vi "TestLidar.vi"() -> ()   [LabVIEW 2018]
uses:
  <vilib>/robotics/Navigation/shared/MapNode/OccupancyGridNode/NI_Robotics_OccupancyGridMapNode.lvclass
  C:/Program Files (x86)/National Instruments/LabVIEW 2018/vi.lib/robotics/Navigation/shared/MapNode/AbstractAstarNode/NI_Robotics_AbstractAstarNode.lvclass
  <vilib>/robotics/Navigation/shared/WorldMap/OccupancyGridWorldMap/NI_Robotics_OccupancyGridWorldMap.lvclass
  C:/Program Files (x86)/National Instruments/LabVIEW 2018/vi.lib/robotics/Navigation/shared/WorldMap/AbstractWorldMap/NI_Robotics_AbstractWorldMap.lvclass
  <vilib>/robotics/Navigation/NI_Robotics_Navigation .lvlib
panel:
  out "Position (mm)":cluster{"X":dbl, "Y":dbl, "Theta":dbl}
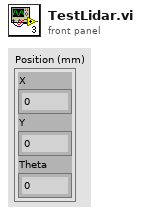
[diagram p1: front panel]
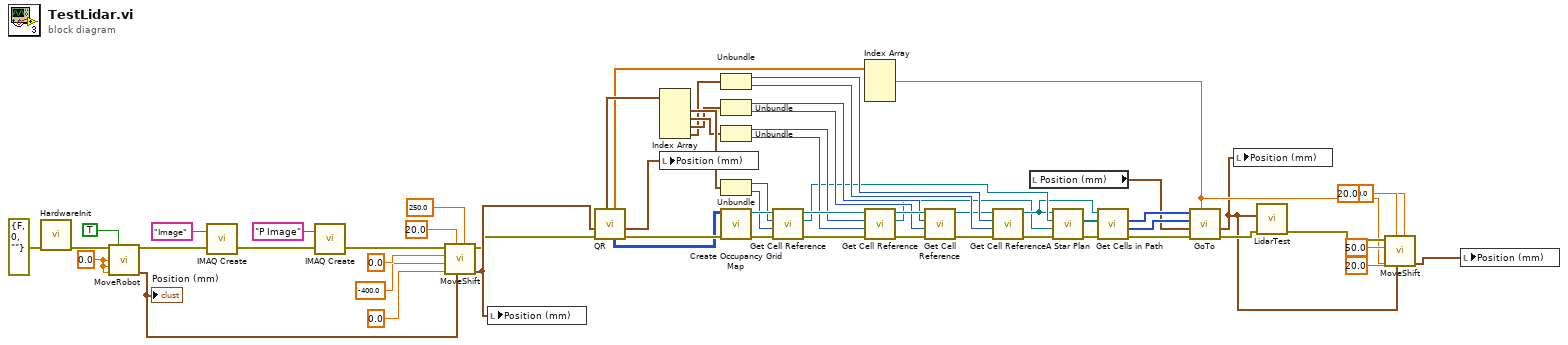
[diagram p0: block diagram]
diagram:
  w59 = 0.0 ("x (mm/s)")
  n1 = call "HardwareInit.vi"("Error/Flow In"=errorcluster {"status"=FALSE, "code"=0, "source"=""}) -> ("error out"=w60:errorcluster)  [unwired: 10 in]
  n2 = call "MoveRobot.vi"("Error/Flow In"=w60, "Reset"=TRUE, "x (mm/s)"=w59, "y (mm/s)"=w59, "theta (rad/s)"=w59) -> ("Error/Flow Out"=w57:errorcluster, "Position"=w47:cluster{"X":dbl, "Y":dbl, "Theta":dbl})  [unwired: 9 in]
  "Position (mm)" <- w47
  n3 = call "IMAQ Create"("Image Name"="Image", "error in (no error)"=w57) -> ("error out"=w55:errorcluster)  [unwired: 3 in, 1 out]
  n4 = call "IMAQ Create"("Image Name"="P Image", "error in (no error)"=w55) -> ("error out"=w53:errorcluster)  [unwired: 3 in, 1 out]
  n5 = call "MoveShift.vi"("max speed"=250.0, "Position"=w47, "Precision"=20.0, "theta"=0.0, "y shift"=-400.0, "x shift"=0.0, "Error/Flow In"=w53) -> ("Position Out"=w46:cluster{"X":dbl, "Y":dbl, "Theta":dbl}, "Error/Flow Out"=w10:errorcluster)  [unwired: 3 in]
  n6 = local write "Position (mm)"(w46) -> ()
  n7 = call "QR.vi"("error in"=w10, "Position"=w46) -> ("error out"=w44:errorcluster, "Position Out"=w45:cluster{"X":dbl, "Y":dbl, "Theta":dbl}, "G"=w43:i32[][], "Control Angles"=w31:dbl[], "Control Points"=w32:cluster{"third_x":i32, "third_y":i32}[])  [unwired: 3 in, 2 out]
  n8 = Index Array(array=w32) -> (element #1=w30:cluster{"third_x":i32, "third_y":i32}, element #2=w27:cluster{"third_x":i32, "third_y":i32}, element #3=w22:cluster{"third_x":i32, "third_y":i32}, element #4=w19:cluster{"third_x":i32, "third_y":i32})  [unwired: 4 in]
  n9 = local write "Position (mm)"(w45) -> ()
  n10 = Unbundle(w19) -> ("third_x"=w18:i32, "third_y"=w17:i32)
  n11 = Unbundle(w22) -> ("third_x"=w21:i32, "third_y"=w20:i32)
  n12 = Unbundle(w27) -> ("third_x"=w26:i32, "third_y"=w25:i32)
  n13 = Unbundle(w30) -> ("third_x"=w29:i32, "third_y"=w28:i32)
  n14 = call <vilib>:"Create Occupancy Grid Map.vi"("error in (no error)"=w44, "occupancy grid"=w43) -> ("error out"=w42:errorcluster, "map reference out"=w41:refnum<data-value>)  [unwired: 8 in]
  n15 = call <vilib>:"Get Cell Reference.vi"("error in (no error)"=w42, "y"=w28, "x"=w29, "map reference in"=w41) -> ("error out"=w39:errorcluster, "cell reference"=w13:refnum<data-value>, "map reference out"=w40:refnum<data-value>)  [unwired: 4 in, 1 out]
  n16 = Index Array(array=w31) -> (element #1=w5:dbl)  [unwired: 3 in, 2 out]
  n17 = call <vilib>:"Get Cell Reference.vi"("error in (no error)"=w39, "y"=w25, "x"=w26, "map reference in"=w40) -> ("error out"=w24:errorcluster, "cell reference"=w11:refnum<data-value>, "map reference out"=w23:refnum<data-value>)  [unwired: 4 in, 1 out]
  n18 = call <vilib>:"Get Cell Reference.vi"("error in (no error)"=w24, "y"=w20, "x"=w21, "map reference in"=w23) -> ("error out"=w15:errorcluster, "map reference out"=w16:refnum<data-value>)  [unwired: 4 in, 2 out]
  n19 = call <vilib>:"Get Cell Reference.vi"("error in (no error)"=w15, "y"=w17, "x"=w18, "map reference in"=w16) -> ("error out"=w14:errorcluster, "map reference out"=w12:refnum<data-value>)  [unwired: 4 in, 2 out]
  n20 = local read "Position (mm)"() -> (w34:cluster{"X":dbl, "Y":dbl, "Theta":dbl})
  n21 = call <vilib>:"A Star Plan.vi"("error in (no error)"=w14, "goal reference"=w11, "start reference"=w13, "map reference in"=w12) -> ("error out"=w38:errorcluster, "path references"=w37:refnum<data-value>[])  [unwired: 4 in, 2 out]
  n22 = call <vilib>:"Get Cells in Path.vi"("error in (no error)"=w38, "path references"=w37, "map reference in"=w12) -> ("error out"=w33:errorcluster, "y coordinates"=w35:i32[], "x coordinates"=w36:i32[])  [unwired: 5 in, 1 out]
  n23 = call "GoTo.vi"("theta"=w5, "error in (no error)"=w33, "Position"=w34, "y path"=w35, "x path"=w36) -> ("Error/Flow Out"=w9:errorcluster, "New Position"=w4:cluster{"X":dbl, "Y":dbl, "Theta":dbl})  [unwired: 5 in]
  n24 = local write "Position (mm)"(w4) -> ()
  n25 = call "LidarTest.vi"("error out"=w9, "Position"=w4) -> ("Error/Flow Out"=w8:errorcluster)  [unwired: 9 in]
  n26 = call "MoveShift.vi"("max speed"=100.0, "Position"=w4, "Precision"=20.0, "theta"=w5, "y shift"=20.0, "x shift"=50.0, "Error/Flow In"=w8) -> ("Position Out"=w3:cluster{"X":dbl, "Y":dbl, "Theta":dbl})  [unwired: 3 in, 1 out]
  n27 = local write "Position (mm)"(w3) -> ()
